vi "Get Dummy Entries.vi"(8 "Error In":errorcluster, 11 "reference in":refnum<class "Electronic Datasheet.lvclass">) -> (0 "Error Out":errorcluster, 2 "Dummy Entries":refnum<class "OD Entry.lvclass">[](array[class]), 3 "reference out":refnum<class "Electronic Datasheet.lvclass">)   [LabVIEW 2024, in "Electronic Datasheet.lvlib" / "Electronic Datasheet.lvclass"]
uses:
  Electronic Datasheet.lvclass
  Core/OD Entry/OD Entry.lvclass
  Core/Dummy Entry/Dummy Entry.lvclass
  D:/git/EDS-File-Viewer/Core/OD Entry/OD Entry.lvclass
  Core/Object Dictionary/Dictionary.lvclass
  Core/OD Section/Section.lvclass
  Core/Value/Value.lvclass
  Core/Electronic Datasheet.lvlib
  Core/Keyname/Key Name.lvclass
  Core/Section Name/Section Name.lvclass
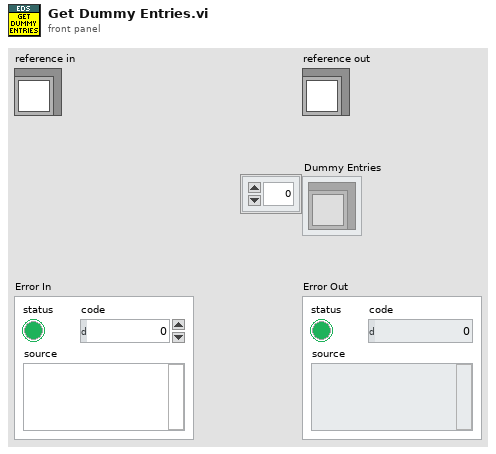
[diagram p1: front panel]
types:
  T1 = typedef "Electronic Datasheet.lvlib/Electronic Datasheet.lvclass/ObjectAttributes.ctl" = cluster{"EDS File Path":path, "Object Dict":refnum<class "Dictionary.lvclass">, "Sorted Object Dict":refnum<class "Sorted Object Dictionary.lvclass">, "Device Info":refnum<class "Device Info.lvclass">, "File Info":refnum<class "File Info.lvclass">}
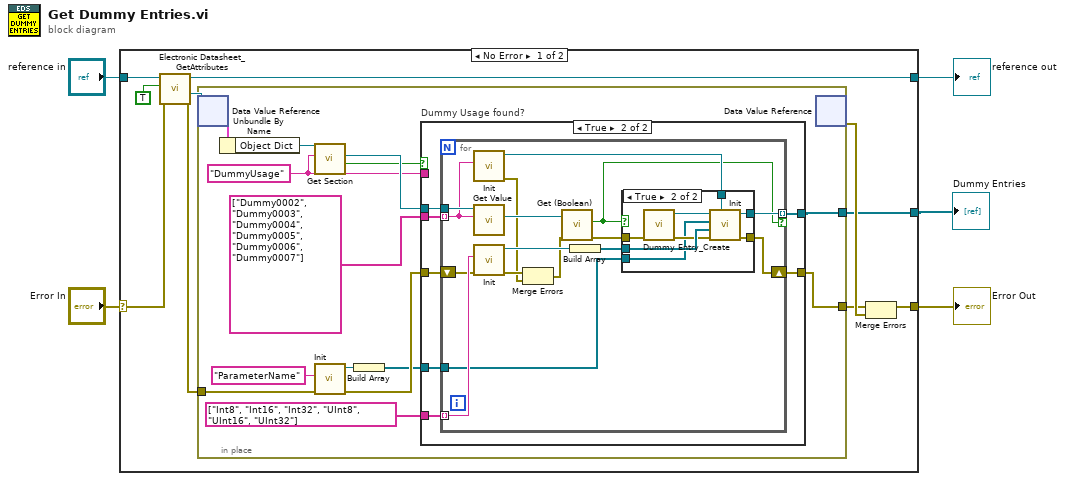
[diagram p0: block diagram]
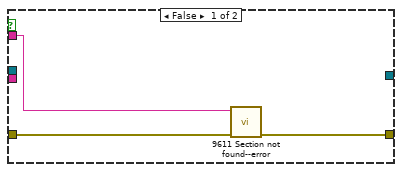
[diagram p2: hidden frame]
diagram:
  n1 = case shown="No Error" "Error In" {
    selector: "Error In" -> [w15 w66]
    tunnel: [w14 w66] -> w4
    tunnel: [w11 w65] -> w2
    tunnel: "reference in" -> [w12 w65]
    tunnel: [w6 _] -> w1
    frame No Error {
      n2 = call "Electronic Datasheet_GetAttributes.vi"("Error In"=w15, "OnlyGetDvrReference(False)"=TRUE, "reference in"=w12) -> ("Error Out"=w8:errorcluster, "DataRef"=w9:refnum<data-value>, "reference out"=w11:refnum<class "Electronic Datasheet.lvclass">)  [unwired: 5 in, 1 out]
      n3 = in-place {
        in-place-border: w8 -> [w20]
        in-place-border: [w23] -> w7
        in-place-border: [w17] -> w6
        w24 = "DummyUsage" ("Section")
        n4 = in-place-dvr #1(w9) -> (w29:T1)  [unwired: 1 out]
        n5 = Unbundle By Name(w29) -> ("Object Dict"=w28:refnum<class "Dictionary.lvclass">)
        n6 = call "Get Section.vi"("Section"=w24, "Dictionary in"=w28) -> ("Found?"=w25:bool, "Section out"=w27:refnum<class "Section.lvclass">)  [unwired: 7 in, 1 out]
        n7 = call "Init.vi"("error in"=w20, "Key Name"="ParameterName") -> ("error out"=w19:errorcluster, "Key Name out"=w18:refnum<class "Key Name.lvclass">)  [unwired: 8 in]
        n8 = Build Array(w18) -> (w16:refnum<class "Key Name.lvclass">[])
        n9 = case "Dummy Usage found?" shown="True" w25 {
          tunnel: w27 -> [_ w39]
          tunnel: string[] ["Dummy0002", "Dummy0003", "Dummy0004", "Dummy0005", "Dummy0006", "Dummy0007"] -> [_ w38]
          tunnel: w19 -> [w32 w37]
          tunnel: [w31 w36] -> w23
          tunnel: w24 -> [w30 _]
          tunnel: [_ w35] -> w17
          tunnel: string[] ["Int8", "Int16", "Int32", "UInt8", "UInt16", "UInt32"] -> [_ w34]
          tunnel: w16 -> [_ w33]
          frame False {
            n10 = call "9611 Section not found--error.vi"("error in (no error)"=w32, "Missing Section Name"=w30) -> ("error out"=w31:errorcluster)  [unwired: 9 in]
          }
          frame True {
            n11 = for {
              tunnel: w39 -> [w52]
              tunnel: w38 -> [w42] mode=indexing
              shift-right: [w53] -> w36
              shift-left: w37 -> [w45]
              tunnel: [w50] -> w35 mode=indexing if=w49
              tunnel: w34 -> [w48] mode=indexing
              tunnel: w33 -> [w47]
              n12 = call "Init.vi"("Section Name"=w42) -> ("error out"=w40:errorcluster, "Section Name out"=w51:refnum<class "Section Name.lvclass">)  [unwired: 9 in]
              n13 = call "Get Value.vi"("Key"=w42, "Object Entry in"=w52) -> ("Value"=w55:refnum<class "Value.lvclass">)  [unwired: 7 in, 2 out]
              n14 = call "Init.vi"("error in"=w45, "Value"=w48) -> ("error out"=w44:errorcluster, "Value out"=w46:refnum<class "Value.lvclass">)  [unwired: 8 in]
              n15 = Merge Errors(w44, w40) -> (w41:errorcluster)
              n16 = call "Get (Boolean).vi"("error in"=w41, "Value in"=w55) -> ("error out"=w54:errorcluster, "Value"=w49:bool)  [unwired: 6 in, 2 out]
              n17 = Build Array(w46) -> (w43:refnum<class "Value.lvclass">[])
              n18 = case shown="True" w49 {
                tunnel: w54 -> [w56 w64]
                tunnel: [w56 w63] -> w53
                tunnel: w51 -> [_ w62]
                tunnel: [_ w61] -> w50
                tunnel: w47 -> [_ w57]
                tunnel: w43 -> [_ w60]
                frame False {
                }
                frame True {
                  n19 = call "Dummy Entry_Create.vi"("Error In"=w64) -> ("Error Out"=w58:errorcluster, "reference out"=w59:refnum<class "Dummy Entry.lvclass">)  [unwired: 9 in]
                  n20 = call-dynamic "Init.vi"("Section Name"=w62, "Error In"=w58, "Values"=w60, "Keys"=w57, "reference in"=w59) -> ("Error Out"=w63:errorcluster, "reference out"=w61:refnum<class "Dummy Entry.lvclass">)  [unwired: 5 in]
                }
              }
            }
          }
        }
        n21 = in-place-dvr #1() -> (w13:errorcluster)  [unwired: 1 in, 1 out]
      }
      n22 = Merge Errors(w7, w13) -> (w14:errorcluster)
    }
    frame Error {
    }
  }
  "Error Out" <- w4
  "reference out" <- w2
  "Dummy Entries" <- w1
